vi "ReadWrite.Data.Commit.vi"(8 "error in":errorcluster, 11 "Ref":T1) -> (0 "error out":errorcluster)   [LabVIEW 2024, in "VS Plugin Data Access Engine.lvlib" / "Plugin Data Access Engine.lvclass"]
uses:
  Plugin Data Access Engine.lvclass
  Types/ReadWrite.DVR.ctl
  Access Type Classes/ReadWrite/ReadWrite.lvclass
  Plugin Data Access Engine.lvclass/Plugin Data Access Engine.ctl
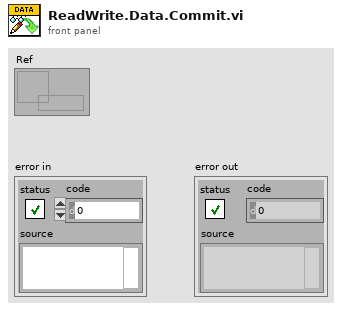
[diagram p1: front panel]
types:
  T1 = typedef "VS Plugin Data Access Engine.lvlib/Plugin Data Access Engine.lvclass/ReadWrite.DVR.ctl" = refnum<data-value>
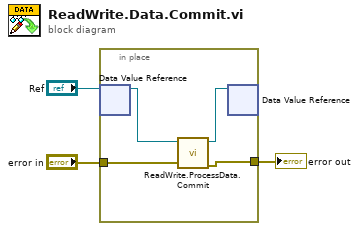
[diagram p0: block diagram]
diagram:
  n1 = in-place {
    in-place-border: "error in" -> [w7]
    in-place-border: [w6] -> w2
    n2 = in-place-dvr #1("Ref") -> (w5:refnum<class "ReadWrite.lvclass">)  [unwired: 1 out]
    n3 = call "ReadWrite.ProcessData.Commit.vi"("error in"=w7, "ReadWrite in"=w5) -> ("error out"=w6:errorcluster, "ReadWrite out"=w4:refnum<class "ReadWrite.lvclass">)  [unwired: 8 in]
    n4 = in-place-dvr #1(w4) -> ()  [unwired: 2 out]
  }
  "error out" <- w2
